vi "Conductus 20C.vi"(2 "Point #":i32, 3 "Instrument Address":refnum<visa-resource-name>) -> (0 "Stop":bool, 1 "Output":dbl[](array[numeric]) format="%.4f")   [LabVIEW 2024]
doc: "This VI reads the sample output of the Lakeshore DRC 93C or 82C temperature controller. The output is an array consisting of the single reading. The input is the numeric GPIB address.\nScott Hannahs, F. Bitter National Magnet Lab, 1993"
panel:
  in  "Sensor":bool
  # "#2"
  # "#1"
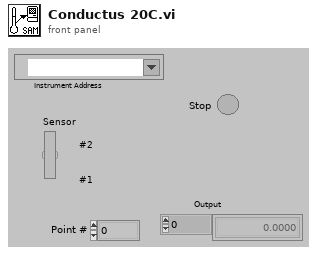
[diagram p1: front panel]
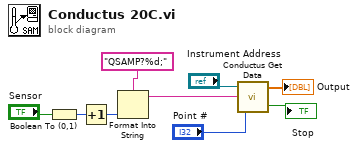
[diagram p0: block diagram]
diagram:
  n1 = Boolean To (0,1)(Boolean="Sensor") -> (0, 1=w4:i16)
  n2 = Increment(x=w4) -> (x+1=w3:i16)
  n3 = Format Into String(format string="QSAMP?%d;", w3) -> (resulting string=w1:string)  [unwired: 2 in, 1 out]
  n4 = call "Conductus Get Data.vi"("Point #"="Point #", "Command String"=w1, "GPIB Address"="Instrument Address") -> ("Stop"=→"Stop":bool, "Measurement"=→"Output":dbl[])
